vi "Image Calibration Mode2.vi"(0 "pObjectImage":u16, 1 "lpszRefPath":string, 2 "nWidth":i32, 3 "nHeight":i32, 4 "nMode":i32, 5 "rectMargin":u32, 6 "bBackGround":i32, 7 "error in (no error)":errorcluster, 8 "lpszDataPath":string, 9 "nAcqMode":i32) -> (18 "lpszDataPath out":string, 20 "pObjectImage out":u16, 21 "lpszRefPath out":string, 22 "function return":i32, 25 "rectMargin out":u32, 27 "error out":errorcluster)   [LabVIEW 2017, in "imgCalibration.lvlib"]
doc: "DLLFunction int __stdcall ImageCalibrationMode2(unsigned short* pObjectImage, LPCTSTR lpszRefPath, int nWidth, int nHeight, int nMode, CRect rectMargin, BOOL bBackGround, LPCTSTR lpszDataPath, int nAcqMode);"
uses:
  imgCalibration.lvlib
  lib/CalibrationDLL.dll
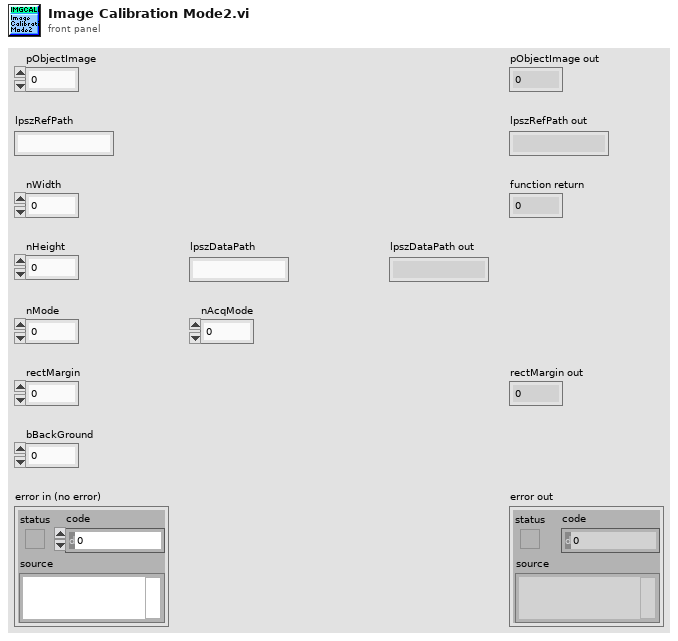
[diagram p1: front panel]
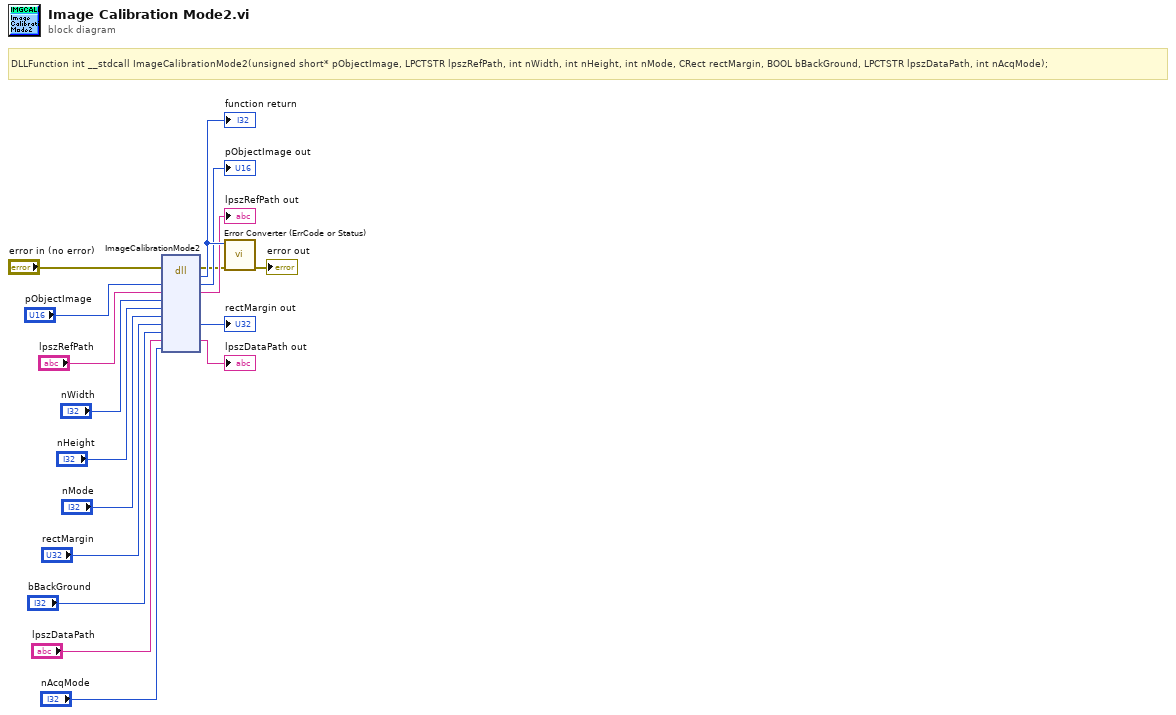
[diagram p0: block diagram]
diagram:
  # "DLLFunction int __stdcall ImageCalibrationMode2(unsigned short* pObjectImage, LPCTSTR lpszRefPath, int nWidth, int nHeight, int nMode, CRect rectMargin, BOOL bBackGround, LPCTSTR lpszDataPath, int nAcqMode);"
  n1 = dll-call lib="F:/BonTechFlatPanelLVDriver/lib/CalibrationDLL.*" fn="ImageCalibrationMode2"(error in="error in (no error)", "pObjectImage"="pObjectImage", "lpszRefPath"="lpszRefPath", "nWidth"="nWidth", "nHeight"="nHeight", "nMode"="nMode", "rectMargin"="rectMargin", "bBackGround"="bBackGround", "lpszDataPath"="lpszDataPath", "nAcqMode"="nAcqMode") -> (error out=w2:errorcluster, w17:i32, "pObjectImage"=→"pObjectImage out":u16, "lpszRefPath"=→"lpszRefPath out":string, "rectMargin"=→"rectMargin out":u32, "lpszDataPath"=→"lpszDataPath out":string)  [unwired: 7 in, 1 out]
  "function return" <- w17
  n2 = call "Error Converter (ErrCode or Status).vi"("error in (no error)"=w2, "error code"=w17) -> ("error out"=→"error out":errorcluster)  [unwired: 9 in]
